vi "ge_XMLTypeDef_toChGrpClass.vi"(8 "error in":errorcluster, 10 "GXML String":string, 11 "ChanGroups":T1) -> (0 "error out":errorcluster, 2 "ChanGrp":refnum<class "ChanGrp.lvclass">[](array[class]))   [LabVIEW 2018]
uses:
  Custom Ctrls/Master CfgXML/ge_XMLHdr_ChanGroups.ctl
  Custom Ctrls/Master Cfg/ge_GrpHdr.ctl
  Custom Ctrls/ge_MeasType.ctl
  Classes/Cfg Grandmaster/Class Chan Group/ChanGrp.lvclass
  Classes/Measurements/Class Voltage/Voltage.lvclass
  C:/Users/Jeff Tipps/Documents/DAQMan/source/Classes/Measurements/Class Channel/Channel.lvclass
  Classes/Cfg Grandmaster/Class Chan Group/Measurement Type Defs/VoltGroup.ctl
  Classes/Cfg Grandmaster/Class Chan Group/Measurement Type Defs/VoltChan.ctl
  Classes/Measurements/Class Channel/ChanProps_TD.ctl
  Classes/Measurements/Class Voltage/VoltProps_TD.ctl
  Classes/Cfg Grandmaster/Class Chan Group/Measurement Type Defs/FreqGroup.ctl
  Classes/Cfg Grandmaster/Class Chan Group/Measurement Type Defs/FreqChan.ctl
  Classes/Measurements/Class Frequency/FreqProps_TD.ctl
  Classes/Measurements/Class Frequency/Frequency.lvclass
  C:/Users/Jeff Tipps/Documents/DAQMan/source/Classes/Measurements/Class Voltage/Voltage.lvclass
  Classes/Cfg Grandmaster/Class Chan Group/Measurement Type Defs/TachGroup.ctl
  Classes/Cfg Grandmaster/Class Chan Group/Measurement Type Defs/TachChan.ctl
  Classes/Measurements/Class Tachometer/TachProps_TD.ctl
  Classes/Measurements/Class Tachometer/Tachometer.lvclass
  C:/Users/Jeff Tipps/Documents/DAQMan/source/Classes/Measurements/Class Frequency/Frequency.lvclass
  Classes/Cfg Grandmaster/Class Chan Group/Measurement Type Defs/DynGroup.ctl
  Classes/Cfg Grandmaster/Class Chan Group/Measurement Type Defs/DyanChan.ctl
  Classes/Measurements/Class Dynamic/DynamicProps_TD.ctl
  Classes/Measurements/Class Dynamic/Dynamic.lvclass
  Classes/Cfg Grandmaster/Class Chan Group/Measurement Type Defs/StrainGroup.ctl
  Classes/Cfg Grandmaster/Class Chan Group/Measurement Type Defs/StrainChan.ctl
  Classes/Measurements/Class Strain/StrainProps_TD.ctl
  Classes/Measurements/Class Strain/Strain.lvclass
  Classes/Cfg Grandmaster/Class Chan Group/Measurement Type Defs/ThrmcplGroup.ctl
  Classes/Cfg Grandmaster/Class Chan Group/Measurement Type Defs/ThrmcplChan.ctl
  Classes/Measurements/Class Thermocouple/ThrmcplProps_TD.ctl
  Classes/Measurements/Class Thermocouple/Thermocouple.lvclass
  Classes/Cfg Grandmaster/Class Chan Group/Measurement Type Defs/RTDGroup.ctl
  Classes/Cfg Grandmaster/Class Chan Group/Measurement Type Defs/RTDChan.ctl
  Classes/Measurements/Class RTD/RTDProps_TD.ctl
  Classes/Measurements/Class RTD/RTD.lvclass
  Classes/Cfg Grandmaster/Class Chan Group/Measurement Type Defs/CurrentGroup.ctl
  Classes/Cfg Grandmaster/Class Chan Group/Measurement Type Defs/CurrentChan.ctl
  Classes/Measurements/Class Current/CurrentProps_TD.ctl
  Classes/Measurements/Class Current/Current.lvclass
  Classes/Cfg Grandmaster/Class Chan Group/Measurement Type Defs/ResGroup.ctl
  Classes/Cfg Grandmaster/Class Chan Group/Measurement Type Defs/ResChan.ctl
  Classes/Measurements/Class Ressistance/ResProps_TD.ctl
  Classes/Measurements/Class Ressistance/Resistance.lvclass
  Classes/Measurements/Class Channel/Channel.lvclass
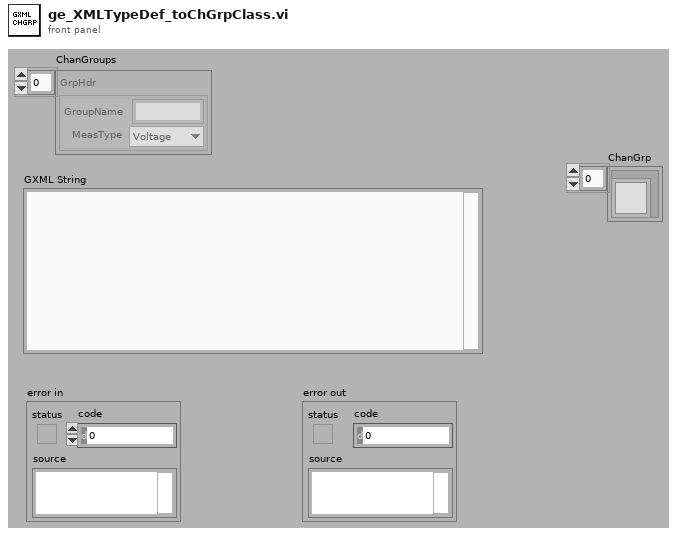
[diagram p1: front panel]
types:
  T1 = typedef "ge_XMLHdr_ChanGroups.ctl" = T2[]
  T2 = typedef "ge_GrpHdr.ctl" = cluster{"GroupName":string, "MeasType":T3}
  T3 = typedef "ge_MeasType.ctl" = enum16{"Voltage", "Frequency", "Tachometer", "Dynamic", "Thermocouple", "RTD", "Strain", "Current", "Resistance"}
  T4 = typedef "Configuration Grandmaster.lvlib/ChanGrp.lvclass/VoltGroup.ctl" = cluster{"GroupName":string, "MeasType":T3, "GroupMems":T5[]}
  T5 = typedef "Configuration Grandmaster.lvlib/ChanGrp.lvclass/VoltChan.ctl" = cluster{"ChanHdr":T6, "VoltChanCfg":T7}
  T6 = typedef "Measurement Channels.lvlib/Channel.lvclass/ChanProps_TD.ctl" = cluster{"ChanName":string, "ModbusAddr":string, "ToModBus":bool, "Alias":string, "Device":string, "Unit_EU":string, "Scale":dbl, "Offset":dbl}
  T7 = typedef "Measurement Channels.lvlib/Voltage.lvclass/VoltProps_TD.ctl" = cluster{"VRange":dbl, "Term Cfg":u16, "Coupling":u16}
  T8 = typedef "Configuration Grandmaster.lvlib/ChanGrp.lvclass/FreqGroup.ctl" = cluster{"GroupName":string, "MeasType":T3, "GroupMems":T9[]}
  T9 = typedef "Configuration Grandmaster.lvlib/ChanGrp.lvclass/FreqChan.ctl" = cluster{"ChanHdr":T6, "VoltChanCfg":T7, "FreqChanCfg":T10}
  T10 = typedef "Measurement Channels.lvlib/Frequency.lvclass/FreqProps_TD.ctl" = cluster{"Thresh":dbl, "Slope":u16, "Min EU":dbl}
  T11 = typedef "Configuration Grandmaster.lvlib/ChanGrp.lvclass/TachGroup.ctl" = cluster{"GroupName":string, "MeasType":T3, "GroupMems":T12[]}
  T12 = typedef "Configuration Grandmaster.lvlib/ChanGrp.lvclass/TachChan.ctl" = cluster{"ChanHdr":T6, "VoltChanCfg":T7, "FreqChanCfg":T10, "TachChanCfg":T13}
  T13 = typedef "Measurement Channels.lvlib/Tachometer.lvclass/TachProps_TD.ctl" = cluster{"PPR":dbl}
  T14 = typedef "Configuration Grandmaster.lvlib/ChanGrp.lvclass/DynGroup.ctl" = cluster{"GroupName":string, "MeasType":T3, "GroupMems":T15[]}
  T15 = typedef "Configuration Grandmaster.lvlib/ChanGrp.lvclass/DyanChan.ctl" = cluster{"ChanHdr":T6, "VoltChanCfg":T7, "DynChanCfg":T16}
  T16 = typedef "Measurement Channels.lvlib/Dynamic.lvclass/DynamicProps_TD.ctl" = cluster{"Sensitivity":dbl, "Iex":dbl, "dB":bool, "dB Ref":dbl, "Cal Mag":dbl, "Cal Units":u16}
  T17 = typedef "Configuration Grandmaster.lvlib/ChanGrp.lvclass/StrainGroup.ctl" = cluster{"GroupName":string, "MeasType":T3, "GroupMems":T18[]}
  T18 = typedef "Configuration Grandmaster.lvlib/ChanGrp.lvclass/StrainChan.ctl" = cluster{"ChanHdr":T6, "StrainChanCfg":T19}
  T19 = typedef "Measurement Channels.lvlib/Strain.lvclass/StrainProps_TD.ctl" = cluster{"Strain Mode":u16, "Vex":dbl, "Bridge Type":u16, "GF":dbl, "Gauge Res":i32, "Poisson":dbl, "Lead Res":dbl, "Init uStrain":dbl, "GAF":dbl, "Approx Max":dbl, "Approx Min":dbl}
  T20 = typedef "Configuration Grandmaster.lvlib/ChanGrp.lvclass/ThrmcplGroup.ctl" = cluster{"GroupName":string, "MeasType":T3, "GroupMems":T21[]}
  T21 = typedef "Configuration Grandmaster.lvlib/ChanGrp.lvclass/ThrmcplChan.ctl" = cluster{"ChanHdr":T6, "ThrmcplChanCfg":T22}
  T22 = typedef "Measurement Channels.lvlib/Thermocouple.lvclass/ThrmcplProps_TD.ctl" = cluster{"Units":u16, "Type":u16, "cjc source":u16, "cjc val":dbl, "Approx Max":dbl, "Approx Min":dbl}
  T23 = typedef "Configuration Grandmaster.lvlib/ChanGrp.lvclass/RTDGroup.ctl" = cluster{"GroupName":string, "MeasType":T3, "GroupMems":T24[]}
  T24 = typedef "Configuration Grandmaster.lvlib/ChanGrp.lvclass/RTDChan.ctl" = cluster{"ChanHdr":T6, "RTDChanCfg":T25}
  T25 = typedef "Measurement Channels.lvlib/RTD.lvclass/RTDProps_TD.ctl" = cluster{"Ro":u16, "Units":u16, "Type":u16, "WireCfg":u16, "Approx Max":dbl, "Approx Min":dbl}
  T26 = typedef "Configuration Grandmaster.lvlib/ChanGrp.lvclass/CurrentGroup.ctl" = cluster{"GroupName":string, "MeasType":T3, "GroupMems":T27[]}
  T27 = typedef "Configuration Grandmaster.lvlib/ChanGrp.lvclass/CurrentChan.ctl" = cluster{"ChanHdr":T6, "CurrentChanCfg":T28}
  T28 = typedef "CurrentProps_TD.ctl" = cluster{"IRange":dbl}
  T29 = typedef "Configuration Grandmaster.lvlib/ChanGrp.lvclass/ResGroup.ctl" = cluster{"GroupName":string, "MeasType":T3, "GroupMems":T30[]}
  T30 = typedef "Configuration Grandmaster.lvlib/ChanGrp.lvclass/ResChan.ctl" = cluster{"ChanHdr":T6, "ResChanCfg":T31}
  T31 = typedef "Measurement Channels.lvlib/Resistance.lvclass/ResProps_TD.ctl" = cluster{"ORange":u16, "WireCfg":u16}
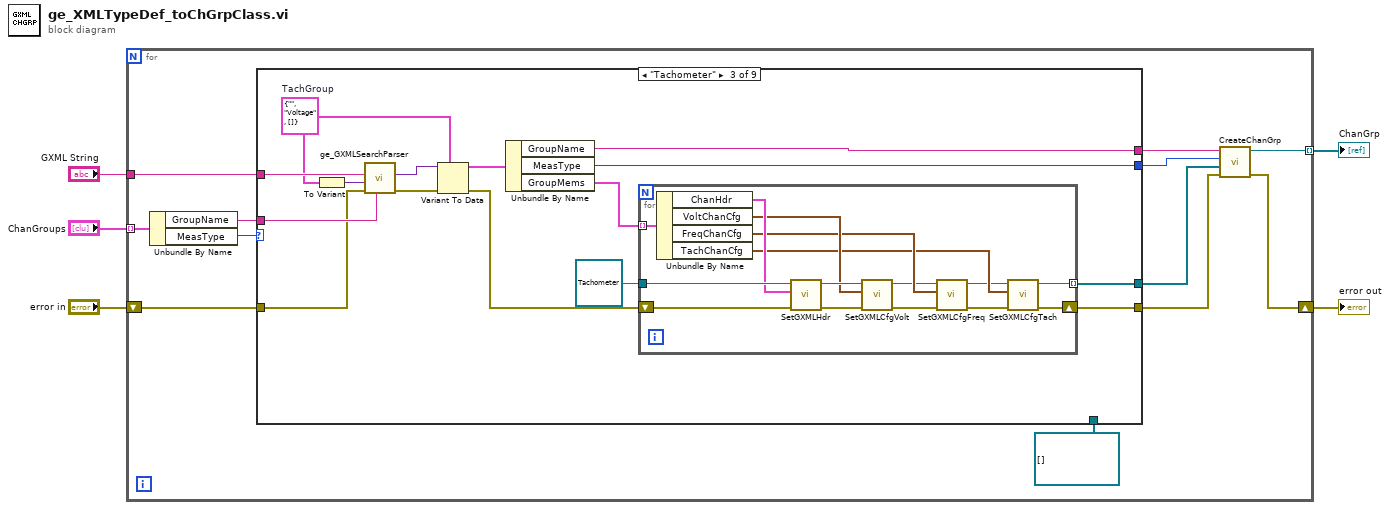
[diagram p0: block diagram]
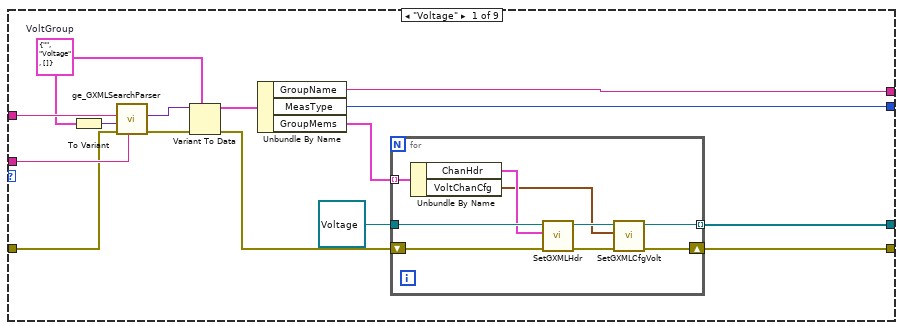
[diagram p2: hidden frame]
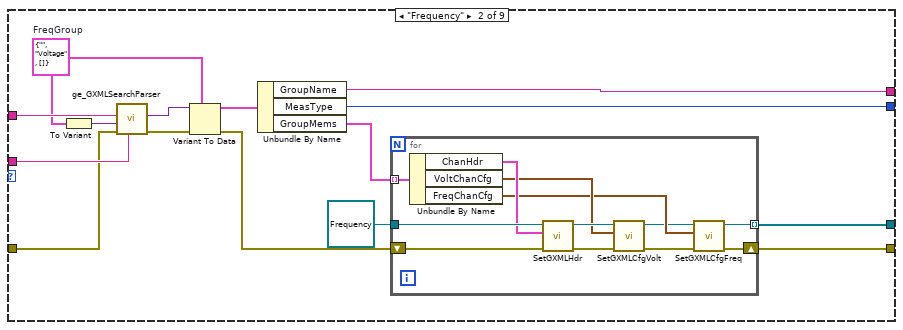
[diagram p3: hidden frame]
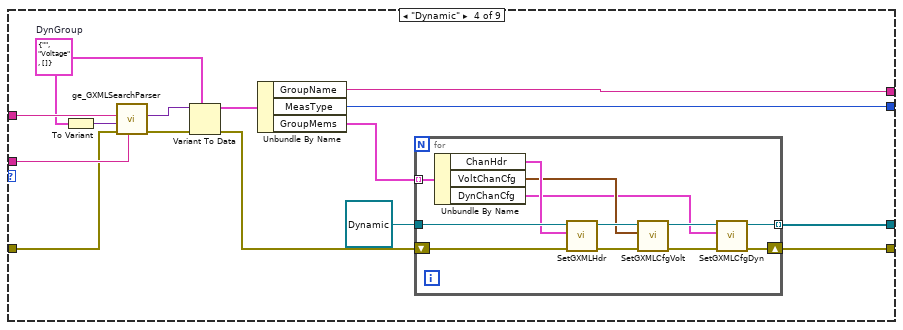
[diagram p4: hidden frame]
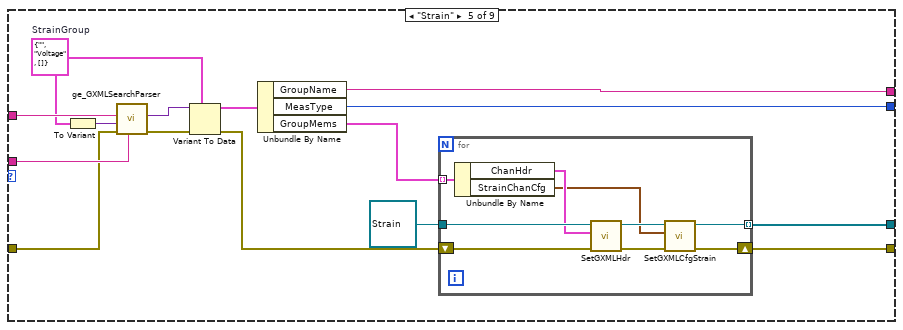
[diagram p5: hidden frame]
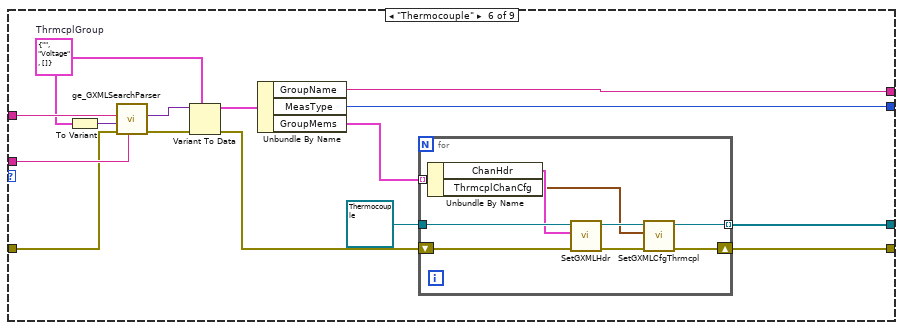
[diagram p6: hidden frame]
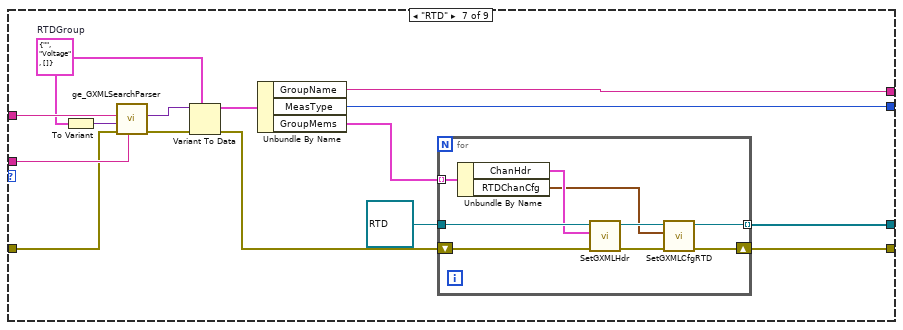
[diagram p7: hidden frame]
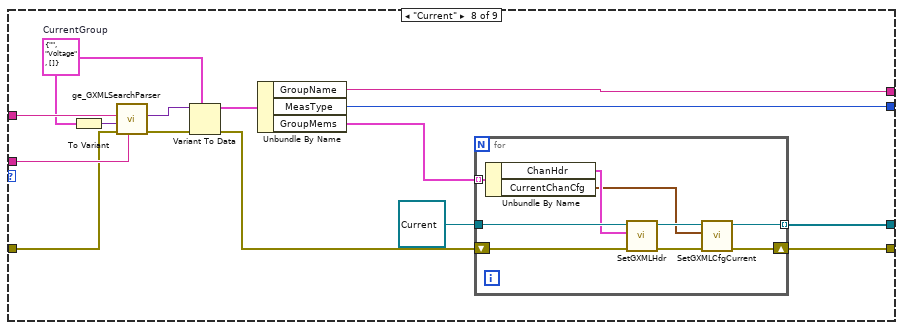
[diagram p8: hidden frame]
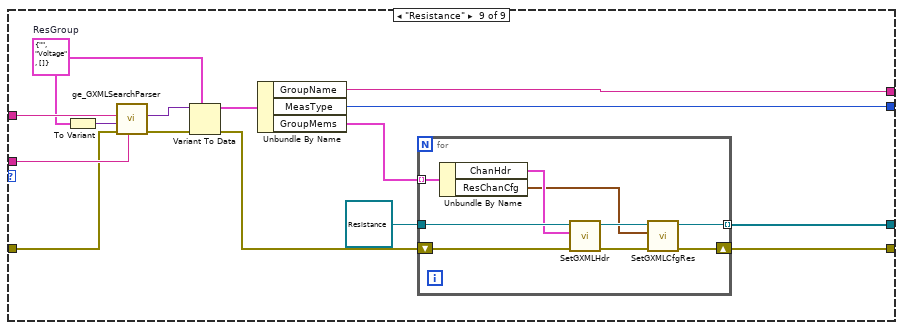
[diagram p9: hidden frame]
diagram:
  n1 = for {
    tunnel: "ChanGroups" -> [w17] mode=indexing
    tunnel: "GXML String" -> [w15]
    shift-right: [w7] -> w5
    shift-left: "error in" -> [w14]
    tunnel: [w6] -> w1 mode=indexing
    n2 = Unbundle By Name(w17) -> ("GroupName"=w16:string, "MeasType"=w13:T3)
    n3 = case shown="\"Tachometer\"" w13 {
      tunnel: w16 -> [w32 w56 w83 w113 w140 w164 w188 w212 w236]
      tunnel: w15 -> [w31 w55 w82 w112 w139 w163 w187 w211 w235]
      tunnel: w14 -> [w30 w54 w81 w111 w138 w162 w186 w210 w234]
      tunnel: [w20 w46 w72 w103 w129 w154 w178 w202 w226] -> w8
      tunnel: [w25 w50 w77 w107 w134 w158 w182 w206 w230] -> w9
      tunnel: [w24 w49 w76 w106 w133 w157 w181 w205 w229] -> w10
      tunnel: [w18 w42 w69 w100 w130 w153 w174 w201 w225] -> w11
      tunnel: refnum<class "Voltage.lvclass">[] [] -> [_ _ _ _ _ _ _ _ _]
      frame "Voltage" {
        w22 = T4 {"GroupName"="", "MeasType"=enum."Voltage", "GroupMems"=[]}  # VoltGroup
        n4 = To Variant(anything=w22) -> (Variant=w23:variant)
        n5 = call "ge_GXMLSearchParser.vi"("String ID"=w32, "error in"=w30, "TypeDesc"=w23, "XML String In"=w31) -> ("error out"=w28:errorcluster, "Parsed Data"=w29:variant)  [unwired: 6 in]
        n6 = Variant To Data(error in=w28, type=w22, Variant=w29) -> (data=w27:T4, error out=w21:errorcluster)
        n7 = Unbundle By Name(w27) -> ("GroupName"=w25:string, "MeasType"=w24:T3, "GroupMems"=w26:T5[])
        n8 = for {
          tunnel: w26 -> [w41] mode=indexing
          tunnel: refnum<class "Voltage.lvclass"> refnum ("Voltage.lvclass") -> [w40]
          shift-right: [w34] -> w20
          shift-left: w21 -> [w38]
          tunnel: [w33] -> w18 mode=indexing
          n9 = Unbundle By Name(w41) -> ("ChanHdr"=w39:T6, "VoltChanCfg"=w35:T7)
          n10 = call "SetGXMLHdr.vi"("error in (no error)"=w38, "ChanHdr"=w39, "Channel in"=w40) -> ("error out"=w37:errorcluster, "Channel out"=w36:refnum<class "Voltage.lvclass">)  [unwired: 7 in]
          n11 = call "SetGXMLCfgVolt.vi"("error in (no error)"=w37, "Voltage Cfg"=w35, "Voltage in"=w36) -> ("error out"=w34:errorcluster, "Voltage out"=w33:refnum<class "Voltage.lvclass">)  [unwired: 7 in]
        }
      }
      frame "Frequency" {
        w47 = T8 {"GroupName"="", "MeasType"=enum."Voltage", "GroupMems"=[]}  # FreqGroup
        n12 = To Variant(anything=w47) -> (Variant=w48:variant)
        n13 = call "ge_GXMLSearchParser.vi"("String ID"=w56, "error in"=w54, "TypeDesc"=w48, "XML String In"=w55) -> ("error out"=w52:errorcluster, "Parsed Data"=w53:variant)  [unwired: 6 in]
        n14 = Variant To Data(error in=w52, type=w47, Variant=w53) -> (data=w51:T8, error out=w45:errorcluster)
        n15 = Unbundle By Name(w51) -> ("GroupName"=w50:string, "MeasType"=w49:T3, "GroupMems"=w44:T9[])
        n16 = for {
          tunnel: w44 -> [w68] mode=indexing
          tunnel: refnum<class "Frequency.lvclass"> refnum ("Frequency.lvclass") -> [w67]
          shift-right: [w58] -> w46
          shift-left: w45 -> [w65]
          tunnel: [w59] -> w42 mode=indexing
          n17 = Unbundle By Name(w68) -> ("ChanHdr"=w66:T6, "VoltChanCfg"=w62:T7, "FreqChanCfg"=w61:T10)
          n18 = call "SetGXMLHdr.vi"("error in (no error)"=w65, "ChanHdr"=w66, "Channel in"=w67) -> ("error out"=w64:errorcluster, "Channel out"=w63:refnum<class "Frequency.lvclass">)  [unwired: 7 in]
          n19 = call "SetGXMLCfgVolt.vi"("error in (no error)"=w64, "Voltage Cfg"=w62, "Voltage in"=w63) -> ("error out"=w57:errorcluster, "Voltage out"=w60:refnum<class "Frequency.lvclass">)  [unwired: 7 in]
          n20 = call "SetGXMLCfgFreq.vi"("error in (no error)"=w57, "FreqChanCfg"=w61, "Freq in"=w60) -> ("error out"=w58:errorcluster, "Freq out"=w59:refnum<class "Frequency.lvclass">)  [unwired: 7 in]
        }
      }
      frame "Tachometer" {
        w74 = T11 {"GroupName"="", "MeasType"=enum."Voltage", "GroupMems"=[]}  # TachGroup
        n21 = To Variant(anything=w74) -> (Variant=w75:variant)
        n22 = call "ge_GXMLSearchParser.vi"("String ID"=w83, "error in"=w81, "TypeDesc"=w75, "XML String In"=w82) -> ("error out"=w79:errorcluster, "Parsed Data"=w80:variant)  [unwired: 6 in]
        n23 = Variant To Data(error in=w79, type=w74, Variant=w80) -> (data=w78:T11, error out=w70:errorcluster)
        n24 = Unbundle By Name(w78) -> ("GroupName"=w77:string, "MeasType"=w76:T3, "GroupMems"=w71:T12[])
        n25 = for {
          tunnel: w71 -> [w98] mode=indexing
          tunnel: refnum<class "Tachometer.lvclass"> refnum ("Tachometer.lvclass") -> [w97]
          shift-right: [w85] -> w72
          shift-left: w70 -> [w95]
          tunnel: [w84] -> w69 mode=indexing
          n26 = Unbundle By Name(w98) -> ("ChanHdr"=w96:T6, "VoltChanCfg"=w92:T7, "FreqChanCfg"=w91:T10, "TachChanCfg"=w88:T13)
          n27 = call "SetGXMLHdr.vi"("error in (no error)"=w95, "ChanHdr"=w96, "Channel in"=w97) -> ("error out"=w94:errorcluster, "Channel out"=w93:refnum<class "Tachometer.lvclass">)  [unwired: 7 in]
          n28 = call "SetGXMLCfgVolt.vi"("error in (no error)"=w94, "Voltage Cfg"=w92, "Voltage in"=w93) -> ("error out"=w89:errorcluster, "Voltage out"=w90:refnum<class "Tachometer.lvclass">)  [unwired: 7 in]
          n29 = call "SetGXMLCfgFreq.vi"("error in (no error)"=w89, "FreqChanCfg"=w91, "Freq in"=w90) -> ("error out"=w86:errorcluster, "Freq out"=w87:refnum<class "Tachometer.lvclass">)  [unwired: 7 in]
          n30 = call "SetGXMLCfgTach.vi"("error in (no error)"=w86, "TachChanCfg"=w88, "Tachometer in"=w87) -> ("error out"=w85:errorcluster, "Tachometer out"=w84:refnum<class "Tachometer.lvclass">)  [unwired: 7 in]
        }
      }
      frame "Dynamic" {
        w104 = T14 {"GroupName"="", "MeasType"=enum."Voltage", "GroupMems"=[]}  # DynGroup
        n31 = To Variant(anything=w104) -> (Variant=w105:variant)
        n32 = call "ge_GXMLSearchParser.vi"("String ID"=w113, "error in"=w111, "TypeDesc"=w105, "XML String In"=w112) -> ("error out"=w109:errorcluster, "Parsed Data"=w110:variant)  [unwired: 6 in]
        n33 = Variant To Data(error in=w109, type=w104, Variant=w110) -> (data=w108:T14, error out=w102:errorcluster)
        n34 = Unbundle By Name(w108) -> ("GroupName"=w107:string, "MeasType"=w106:T3, "GroupMems"=w99:T15[])
        n35 = for {
          tunnel: w99 -> [w125] mode=indexing
          tunnel: refnum<class "Dynamic.lvclass"> refnum ("Dynamic.lvclass") -> [w124]
          shift-right: [w115] -> w103
          shift-left: w102 -> [w122]
          tunnel: [w114] -> w100 mode=indexing
          n36 = Unbundle By Name(w125) -> ("ChanHdr"=w123:T6, "VoltChanCfg"=w119:T7, "DynChanCfg"=w117:T16)
          n37 = call "SetGXMLHdr.vi"("error in (no error)"=w122, "ChanHdr"=w123, "Channel in"=w124) -> ("error out"=w121:errorcluster, "Channel out"=w120:refnum<class "Dynamic.lvclass">)  [unwired: 7 in]
          n38 = call "SetGXMLCfgVolt.vi"("error in (no error)"=w121, "Voltage Cfg"=w119, "Voltage in"=w120) -> ("error out"=w116:errorcluster, "Voltage out"=w118:refnum<class "Dynamic.lvclass">)  [unwired: 7 in]
          n39 = call "SetGXMLCfgDyn.vi"("error in (no error)"=w116, "DynChanCfg"=w117, "Dynamic in"=w118) -> ("error out"=w115:errorcluster, "Dynamic out"=w114:refnum<class "Dynamic.lvclass">)  [unwired: 7 in]
        }
      }
      frame "Strain" {
        w131 = T17 {"GroupName"="", "MeasType"=enum."Voltage", "GroupMems"=[]}  # StrainGroup
        n40 = To Variant(anything=w131) -> (Variant=w132:variant)
        n41 = call "ge_GXMLSearchParser.vi"("String ID"=w140, "error in"=w138, "TypeDesc"=w132, "XML String In"=w139) -> ("error out"=w136:errorcluster, "Parsed Data"=w137:variant)  [unwired: 6 in]
        n42 = Variant To Data(error in=w136, type=w131, Variant=w137) -> (data=w135:T17, error out=w128:errorcluster)
        n43 = Unbundle By Name(w135) -> ("GroupName"=w134:string, "MeasType"=w133:T3, "GroupMems"=w127:T18[])
        n44 = for {
          tunnel: w127 -> [w149] mode=indexing
          tunnel: refnum<class "Strain.lvclass"> refnum ("Strain.lvclass") -> [w148]
          shift-right: [w142] -> w129
          shift-left: w128 -> [w146]
          tunnel: [w144] -> w130 mode=indexing
          n45 = Unbundle By Name(w149) -> ("ChanHdr"=w147:T6, "StrainChanCfg"=w141:T19)
          n46 = call "SetGXMLHdr.vi"("error in (no error)"=w146, "ChanHdr"=w147, "Channel in"=w148) -> ("error out"=w143:errorcluster, "Channel out"=w145:refnum<class "Strain.lvclass">)  [unwired: 7 in]
          n47 = call "SetGXMLCfgStrain.vi"("error in (no error)"=w143, "StrainChanCfg"=w141, "Strain in"=w145) -> ("error out"=w142:errorcluster, "Strain out"=w144:refnum<class "Strain.lvclass">)  [unwired: 7 in]
        }
      }
      frame "Thermocouple" {
        w155 = T20 {"GroupName"="", "MeasType"=enum."Voltage", "GroupMems"=[]}  # ThrmcplGroup
        n48 = To Variant(anything=w155) -> (Variant=w156:variant)
        n49 = call "ge_GXMLSearchParser.vi"("String ID"=w164, "error in"=w162, "TypeDesc"=w156, "XML String In"=w163) -> ("error out"=w160:errorcluster, "Parsed Data"=w161:variant)  [unwired: 6 in]
        n50 = Variant To Data(error in=w160, type=w155, Variant=w161) -> (data=w159:T20, error out=w152:errorcluster)
        n51 = Unbundle By Name(w159) -> ("GroupName"=w158:string, "MeasType"=w157:T3, "GroupMems"=w151:T21[])
        n52 = for {
          tunnel: w151 -> [w173] mode=indexing
          tunnel: refnum<class "Thermocouple.lvclass"> refnum ("Thermocouple.lvclass") -> [w172]
          shift-right: [w165] -> w154
          shift-left: w152 -> [w170]
          tunnel: [w168] -> w153 mode=indexing
          n53 = Unbundle By Name(w173) -> ("ChanHdr"=w171:T6, "ThrmcplChanCfg"=w167:T22)
          n54 = call "SetGXMLHdr.vi"("error in (no error)"=w170, "ChanHdr"=w171, "Channel in"=w172) -> ("error out"=w166:errorcluster, "Channel out"=w169:refnum<class "Thermocouple.lvclass">)  [unwired: 7 in]
          n55 = call "SetGXMLCfgThrmcpl.vi"("error in (no error)"=w166, "ThrmcplChanCfg"=w167, "Thermocouple in"=w169) -> ("error out"=w165:errorcluster, "Thermocouple out"=w168:refnum<class "Thermocouple.lvclass">)  [unwired: 7 in]
        }
      }
      frame "RTD" {
        w179 = T23 {"GroupName"="", "MeasType"=enum."Voltage", "GroupMems"=[]}  # RTDGroup
        n56 = To Variant(anything=w179) -> (Variant=w180:variant)
        n57 = call "ge_GXMLSearchParser.vi"("String ID"=w188, "error in"=w186, "TypeDesc"=w180, "XML String In"=w187) -> ("error out"=w184:errorcluster, "Parsed Data"=w185:variant)  [unwired: 6 in]
        n58 = Variant To Data(error in=w184, type=w179, Variant=w185) -> (data=w183:T23, error out=w177:errorcluster)
        n59 = Unbundle By Name(w183) -> ("GroupName"=w182:string, "MeasType"=w181:T3, "GroupMems"=w176:T24[])
        n60 = for {
          tunnel: w176 -> [w197] mode=indexing
          tunnel: refnum<class "RTD.lvclass"> refnum ("RTD.lvclass") -> [w196]
          shift-right: [w190] -> w178
          shift-left: w177 -> [w194]
          tunnel: [w189] -> w174 mode=indexing
          n61 = Unbundle By Name(w197) -> ("ChanHdr"=w195:T6, "RTDChanCfg"=w192:T25)
          n62 = call "SetGXMLHdr.vi"("error in (no error)"=w194, "ChanHdr"=w195, "Channel in"=w196) -> ("error out"=w191:errorcluster, "Channel out"=w193:refnum<class "RTD.lvclass">)  [unwired: 7 in]
          n63 = call "SetGXMLCfgRTD.vi"("error in (no error)"=w191, "RTDChanCfg"=w192, "RTD in"=w193) -> ("error out"=w190:errorcluster, "RTD out"=w189:refnum<class "RTD.lvclass">)  [unwired: 7 in]
        }
      }
      frame "Current" {
        w203 = T26 {"GroupName"="", "MeasType"=enum."Voltage", "GroupMems"=[]}  # CurrentGroup
        n64 = To Variant(anything=w203) -> (Variant=w204:variant)
        n65 = call "ge_GXMLSearchParser.vi"("String ID"=w212, "error in"=w210, "TypeDesc"=w204, "XML String In"=w211) -> ("error out"=w208:errorcluster, "Parsed Data"=w209:variant)  [unwired: 6 in]
        n66 = Variant To Data(error in=w208, type=w203, Variant=w209) -> (data=w207:T26, error out=w200:errorcluster)
        n67 = Unbundle By Name(w207) -> ("GroupName"=w206:string, "MeasType"=w205:T3, "GroupMems"=w199:T27[])
        n68 = for {
          tunnel: w199 -> [w221] mode=indexing
          tunnel: refnum<class "Current.lvclass"> refnum ("Current.lvclass") -> [w220]
          shift-right: [w214] -> w202
          shift-left: w200 -> [w218]
          tunnel: [w213] -> w201 mode=indexing
          n69 = Unbundle By Name(w221) -> ("ChanHdr"=w219:T6, "CurrentChanCfg"=w216:T28)
          n70 = call "SetGXMLHdr.vi"("error in (no error)"=w218, "ChanHdr"=w219, "Channel in"=w220) -> ("error out"=w215:errorcluster, "Channel out"=w217:refnum<class "Current.lvclass">)  [unwired: 7 in]
          n71 = call "SetGXMLCfgCurrent.vi"("error in (no error)"=w215, "CurrentChanCfg"=w216, "Current in"=w217) -> ("error out"=w214:errorcluster, "Current out"=w213:refnum<class "Current.lvclass">)  [unwired: 7 in]
        }
      }
      frame "Resistance" {
        w227 = T29 {"GroupName"="", "MeasType"=enum."Voltage", "GroupMems"=[]}  # ResGroup
        n72 = To Variant(anything=w227) -> (Variant=w228:variant)
        n73 = call "ge_GXMLSearchParser.vi"("String ID"=w236, "error in"=w234, "TypeDesc"=w228, "XML String In"=w235) -> ("error out"=w232:errorcluster, "Parsed Data"=w233:variant)  [unwired: 6 in]
        n74 = Variant To Data(error in=w232, type=w227, Variant=w233) -> (data=w231:T29, error out=w224:errorcluster)
        n75 = Unbundle By Name(w231) -> ("GroupName"=w230:string, "MeasType"=w229:T3, "GroupMems"=w223:T30[])
        n76 = for {
          tunnel: w223 -> [w245] mode=indexing
          tunnel: refnum<class "Resistance.lvclass"> refnum ("Resistance.lvclass") -> [w244]
          shift-right: [w238] -> w226
          shift-left: w224 -> [w242]
          tunnel: [w240] -> w225 mode=indexing
          n77 = Unbundle By Name(w245) -> ("ChanHdr"=w243:T6, "ResChanCfg"=w237:T31)
          n78 = call "SetGXMLHdr.vi"("error in (no error)"=w242, "ChanHdr"=w243, "Channel in"=w244) -> ("error out"=w239:errorcluster, "Channel out"=w241:refnum<class "Resistance.lvclass">)  [unwired: 7 in]
          n79 = call "SetGXMLCfgRes.vi"("error in (no error)"=w239, "ResChanCfg"=w237, "Resistance in"=w241) -> ("error out"=w238:errorcluster, "Resistance out"=w240:refnum<class "Resistance.lvclass">)  [unwired: 7 in]
        }
      }
    }
    n80 = call "CreateChanGrp.vi"("error in (no error)"=w8, "GroupChans"=w11, "MeasType"=w10, "GroupName"=w9) -> ("error out"=w7:errorcluster, "ChanGrp out"=w6:refnum<class "ChanGrp.lvclass">)  [unwired: 6 in]
  }
  "error out" <- w5
  "ChanGrp" <- w1
